vi "Module Stopping.vi"(8 "error in":errorcluster) -> (0 "error out":errorcluster)   [LabVIEW 2015, in "Generic Module Library.lvlib" / "Template G_Module.lvlib"]
uses:
  Template G_Module.lvlib
  Private Controls/Event Item.ctl
  Broadcast Support/Broadcast Actions.ctl
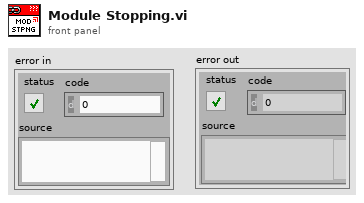
[diagram p1: front panel]
types:
  T1 = typedef "Generic Module Library.lvlib/Template G_Module.lvlib/Broadcast Actions.ctl" = enum16{"Create", "Get", "Destroy"}
  T2 = typedef "Generic Module Library.lvlib/Template G_Module.lvlib/Event Item.ctl" = cluster{"Event Data":variant}
  T3 = typedef "Generic Module Library.lvlib/Template G_Module.lvlib/Broadcast List.ctl" = cluster{"Module Started":refnum<user-event>, "Module Error":refnum<user-event>, "Module Pong":refnum<user-event>, "Module Status":refnum<user-event>, "Module Stopping":refnum<user-event>, "Module Stopped":refnum<user-event>, "Module Reinitialized":refnum<user-event>}
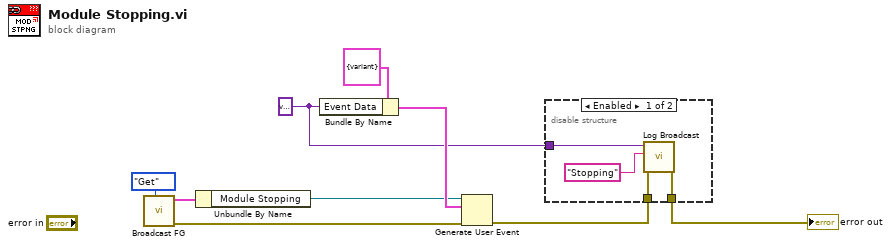
[diagram p0: block diagram]
diagram:
  w3 = variant ("Broadcast Data")
  n1 = call "Broadcast FG.vi"("Broadcast Actions"=Broadcast_Actions."Get") -> ("error out"=w9:errorcluster, "Broadcast List"=w4:T3)  [unwired: 9 in]
  n2 = Unbundle By Name(w4) -> ("Module Stopping"=w5:refnum<user-event>)
  n3 = Bundle By Name(cluster=T2 {"Event Data"=variant} ("Broadcast Item"), "Event Data"=w3) -> (w7:T2)
  n4 = Generate User Event(user event=w5, event data cluster=w7, error in=w9) -> (error out=w2:errorcluster)  [unwired: 1 in, 1 out]
  n5 = disable-structure shown="Enabled" {
    disable-tunnel: w2 -> [w13 w14]
    disable-tunnel: [w12 w14] -> w1
    disable-tunnel: w3 -> [w10 _]
    frame Enabled {
      n6 = call "Log Broadcast.vi"("error in"=w13, "Broadcast Name"="Stopping", "Message Data In"=w10) -> ("error out"=w12:errorcluster)  [unwired: 8 in]
    }
    frame Disabled {
    }
  }
  "error out" <- w1
